vi "Регулятор.vi"() -> ()   [LabVIEW 2021]
panel:
  in  "I":dbl
  in  "PrevErr":dbl
  in  "Температура\nснаружи":dbl
  in  "Температура\nдома":dbl
  in  "Установить\nтемпературу":dbl
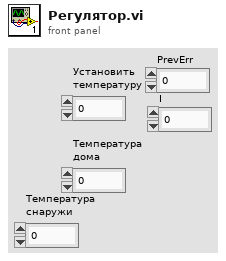
[diagram p1: front panel]
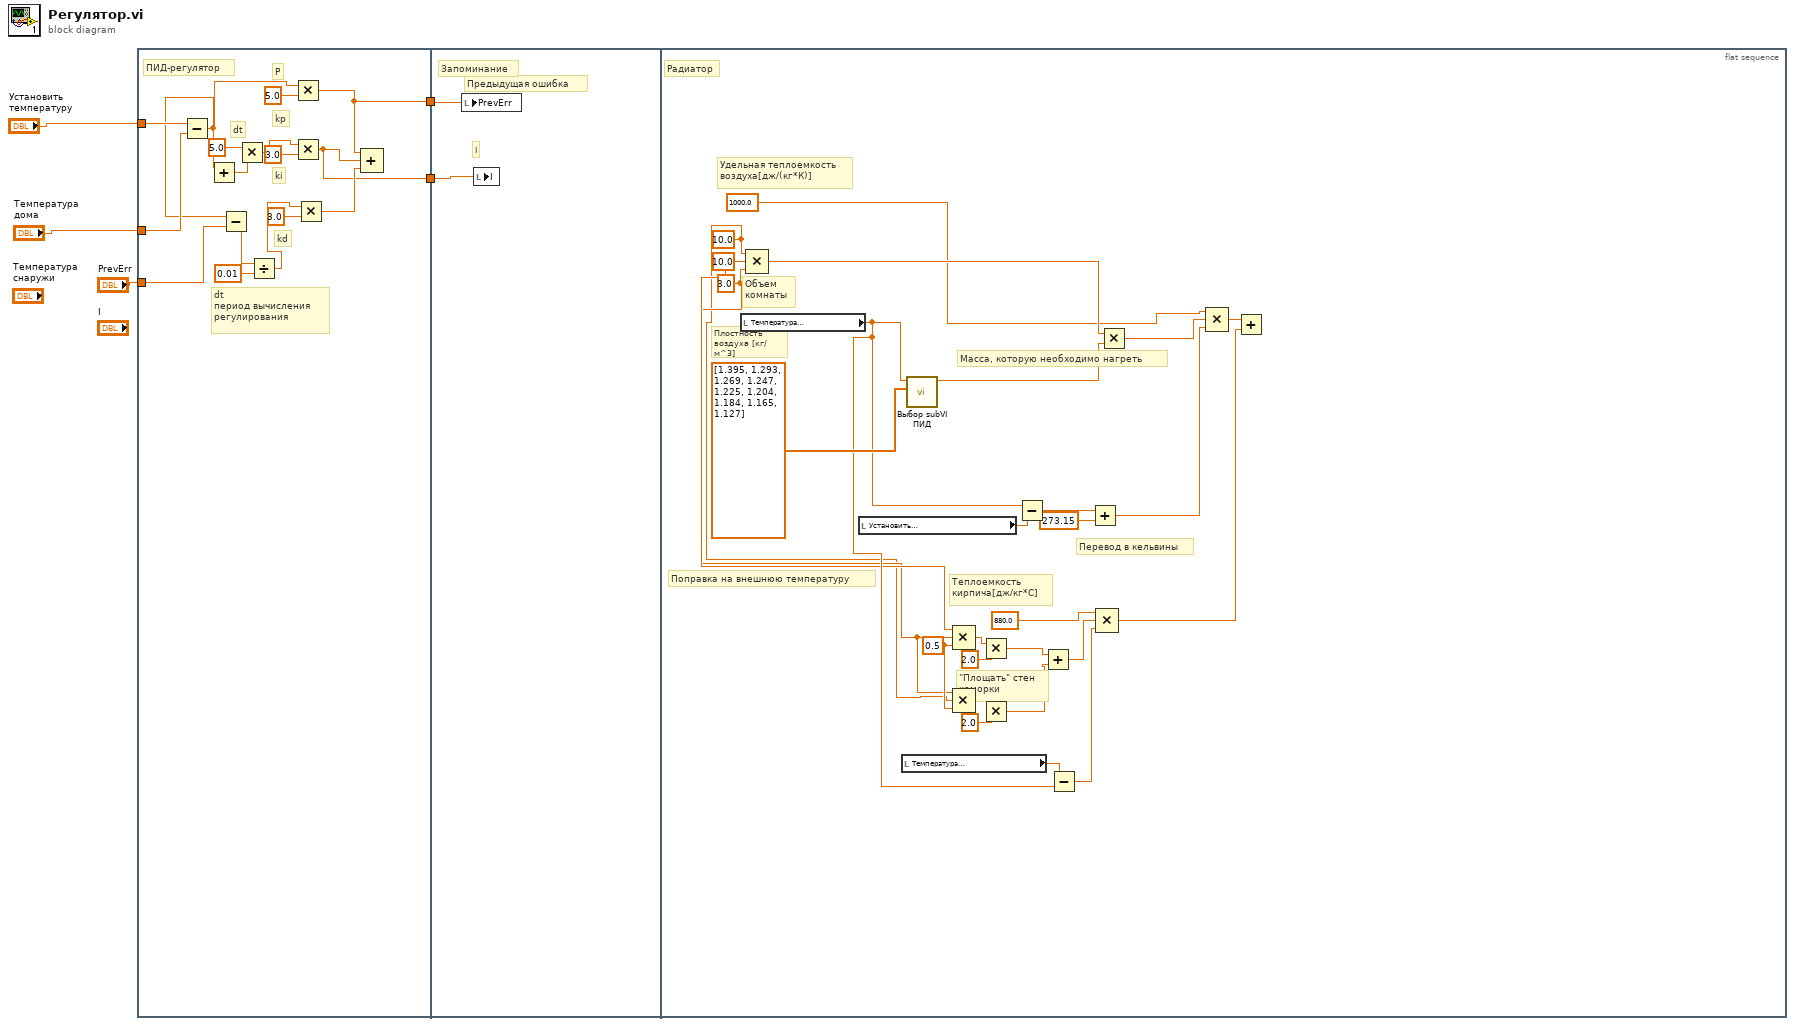
[diagram p0: block diagram]
diagram:
  n1 = flat-sequence {
    tunnel: [w12] -> w5
    tunnel: [w6] -> w4
    tunnel: "Установить\nтемпературу" -> [w18]
    tunnel: "Температура\nдома" -> [w16]
    tunnel: "PrevErr" -> [w7]
    tunnel: w5 -> [w22]
    tunnel: w4 -> [w23]
    frame #0 {
      # "ПИД-регулятор"
      # "dt\nпериод вычисления \nрегулирования"
      # "dt"
      # "P"
      # "kd"
      # "ki"
      # "kp"
      n2 = Subtract(x=w18, y=w16) -> (x-y=w11:dbl)
      n3 = Add(x=w11) -> (x+y=w15:dbl)  [unwired: 1 in]
      n4 = Subtract(x=w11, y=w7) -> (x-y=w10:dbl)
      n5 = Multiply(x=5.0, y=w15) -> (x*y=w13:dbl)
      n6 = Divide(x=w10, y=0.01) -> (x/y=w8:dbl)
      n7 = Multiply(x=w11, y=5.0) -> (x*y=w12:dbl)
      n8 = Multiply(x=w13, y=3.0) -> (x*y=w6:dbl)
      n9 = Multiply(x=w8, y=3.0) -> (x*y=w17:dbl)
      n10 = Compound Arithmetic op=ADD(w12, w6, w17) -> ()  [unwired: 1 out]
    }
    frame #1 {
      # "Запоминание"
      # "I"
      # "Предыдущая ошибка"
      n11 = local write "PrevErr"(w22) -> ()
      n12 = local write "I"(w23) -> ()
    }
    frame #2 {
      w31 = 0.5 ("value")
      w35 = 10.0 ("value")
      w30 = 3.0 ("value")
      w29 = 10.0 ("value")
      # "\"Площать\" стен\nкоморки"
      # "Теплоемкость\nкирпича[дж/кг*С]"
      # "Поправка на внешнюю температуру"
      # "Перевод в кельвины"
      # "Удельная теплоемкость\nвоздуха[дж/(кг*К)]"
      # "Масса, которую необходимо нагреть"
      # "Плостность \nвоздуха [кг/м^3]"
      # "Радиатор"
      # "Объем \nкомнаты"
      n13 = local read "Температура\nдома"() -> (w38:dbl)
      n14 = Compound Arithmetic op=MULTIPLY(w29, w35, w30) -> (w46:dbl)
      n15 = local read "Установить\nтемпературу"() -> (w43:dbl)
      n16 = local read "Температура\nснаружи"() -> (w39:dbl)
      n17 = call "Выбор subVI ПИД.vi"("Array"=dbl[] [1.395, 1.293, 1.269, 1.247, 1.225, 1.204, 1.184, 1.165, 1.127], "Температура\nдома"=w38) -> ("Numeric"=w47:dbl)  [unwired: 9 in]
      n18 = Compound Arithmetic op=MULTIPLY(w35, w30, w31) -> (w34:dbl)
      n19 = Compound Arithmetic op=MULTIPLY(w30, w29, w31) -> ()  [unwired: 1 out]
      n20 = Multiply(x=w34, y=2.0) -> (x*y=w28:dbl)
      n21 = Multiply(y=2.0) -> (x*y=w27:dbl)  [unwired: 1 in]
      n22 = Subtract(x=w38, y=w43) -> (x-y=w42:dbl)
      n23 = Add(x=w28, y=w27) -> (x+y=w26:dbl)
      n24 = Subtract(x=w39, y=w38) -> (x-y=w37:dbl)
      n25 = Add(x=w42, y=273.15) -> (x+y=w40:dbl)
      n26 = Compound Arithmetic op=MULTIPLY(880.0 ("value"), w26, w37) -> (w24:dbl)
      n27 = Multiply(x=w46, y=w47) -> (x*y=w44:dbl)
      n28 = Compound Arithmetic op=MULTIPLY(1000.0 ("value"), w44, w40) -> (w25:dbl)
      n29 = Add(x=w25, y=w24) -> ()  [unwired: 1 out]
    }
  }
